vi "acqComponentsInit.vi"(1 "sCMOS init":cluster{"init":i16, "sCMOS handle":u32}, 2 "XY stage":T5, 3 "Z stage":T4, 4 "Filter wheel init":cluster{"FW Handle":u32, "init?":i16}, 6 "405 nm (aq)":bool=TRUE, 7 "405 nm filter":T3(ring), 8 "488 nm (aq)":bool=TRUE, 9 "488 nm filter":T3(ring)=enum."525/50 [FITC]", 10 "561 nm (aq)":bool=TRUE, 11 "561 nm filter":T3(ring)=enum."605/70 [Cy3]", 12 "642 nm (aq)":bool=TRUE, 13 "642 nm filter":T3(ring)=enum."665/LP [Cy5]") -> (15 "initializedLasers":T1(array[cluster]), 16 "Initialized filters":T2(array[ring])=[enum."460/36 [DAPI]", enum."525/50 [FITC]", enum."605/70 [Cy3]", enum."665/LP [Cy5]"], 17 "correctCompInit?":i32)   [LabVIEW 2015]
panel:
  in  "LSFM_3 lasers":T1(array[cluster])=[{"Component ID"="405nm", "COM Port"="COM14", "Type "=enum."omicronLuxX", "init"=1}, {"Component ID"="488nm", "COM Port"="COM4", "Type "=enum."omicronLuxX", "init"=1}, {"Component ID"="561nm", "COM Port"="COM27", "Type "=enum."coherentObis", "init"=1}, {"Component ID"="642nm", "COM Port"="COM12", "Type "=enum."omicronLuxX", "init"=1}]
  out "Correct lasers init?":i32=1
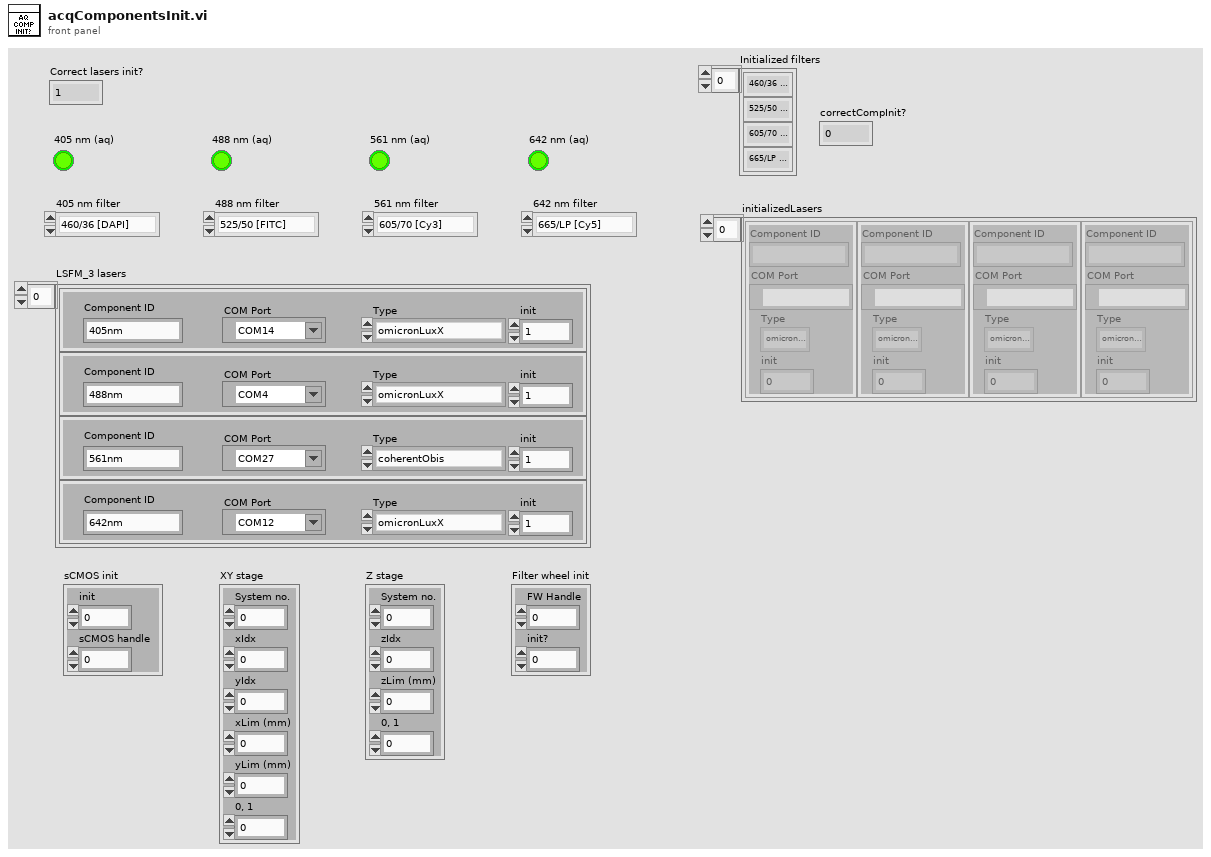
[diagram p1: front panel]
types:
  T1 = cluster{"Component ID":string, "COM Port":refnum<visa-resource-name>, "Type ":enum16{"omicronLuxX", "coherentObis"}, "init":i16}[]
  T2 = enum16{"460/36 [DAPI]", "525/50 [FITC]", "605/70 [Cy3]", "665/LP [Cy5]", "Empty-1", "Empty-2"}[]
  T3 = enum16{"460/36 [DAPI]", "525/50 [FITC]", "605/70 [Cy3]", "665/LP [Cy5]", "Empty-1", "Empty-2"}
  T4 = cluster{"System no.":i32, "zIdx":i32, "zLim (mm)":dbl, "0, 1":i16}
  T5 = cluster{"System no.":i32, "xIdx":i32, "yIdx":i32, "xLim (mm)":dbl, "yLim (mm)":dbl, "0, 1":i16}
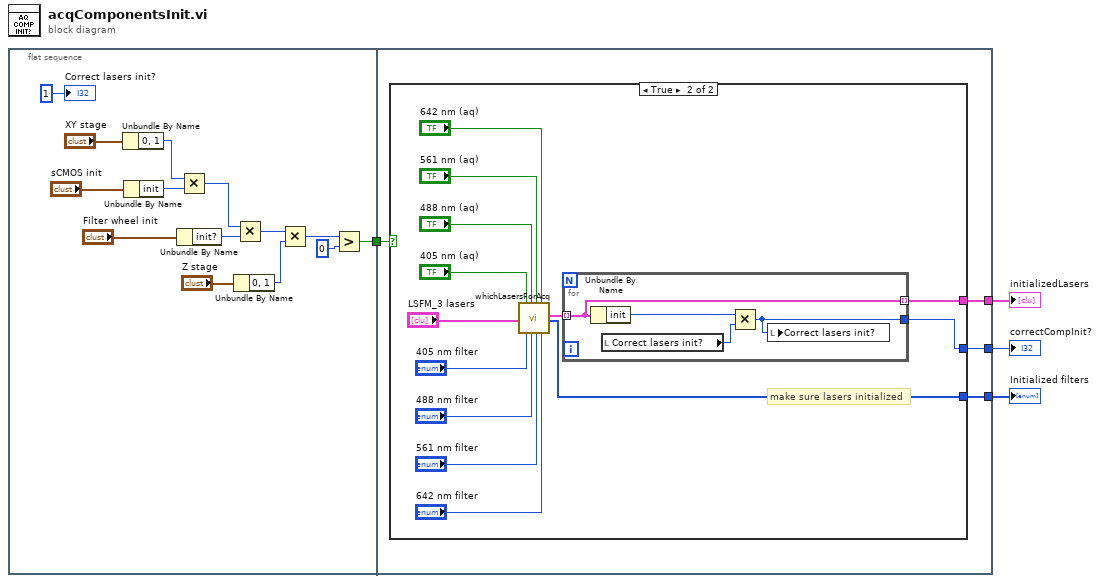
[diagram p0: block diagram]
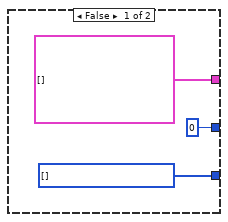
[diagram p2: hidden frame]
diagram:
  n1 = flat-sequence {
    tunnel: [w5] -> w1
    tunnel: [w22] -> w4
    tunnel: [w21] -> w3
    tunnel: [w20] -> w2
    tunnel: w1 -> [w19]
    frame #0 {
      n2 = Unbundle By Name("XY stage") -> ("0, 1"=w13:i16)
      n3 = Unbundle By Name("sCMOS init") -> ("init"=w12:i16)
      n4 = Unbundle By Name("Filter wheel init") -> ("init?"=w10:i16)
      n5 = Multiply(x=w13, y=w12) -> (x*y=w11:i16)
      n6 = Unbundle By Name("Z stage") -> ("0, 1"=w8:i16)
      n7 = Multiply(x=w11, y=w10) -> (x*y=w9:i16)
      n8 = Multiply(x=w9, y=w8) -> (x*y=w6:i16)
      n9 = Greater?(x=w6, y=0) -> (0:w5:bool)
      "Correct lasers init?" <- 1 ("Correct lasers init?")
    }
    frame #1 {
      n10 = case shown="True" w19 {
        tunnel: [0 w28] -> w22
        tunnel: [T1 [] w27] -> w21
        tunnel: [w23 w26] -> w20
        frame False {
          w23 = T2 [] items=["460/36 [DAPI]", "525/50 [FITC]", "605/70 [Cy3]", "665/LP [Cy5]", "Empty-1", "Empty-2"] ("Array 2")
        }
        frame True {
          # "make sure lasers initialized"
          n11 = call "whichLasersForAcq.vi"("LSFM_3 lasers"="LSFM_3 lasers", "405 nm (aq)"="405 nm (aq)", "405 nm filter"="405 nm filter", "488 nm (aq)"="488 nm (aq)", "488 nm filter"="488 nm filter", "561 nm (aq)"="561 nm (aq)", "561 nm filter"="561 nm filter", "642 nm (aq)"="642 nm (aq)", "642 nm filter"="642 nm filter") -> ("Initialized lasers"=w38:T1, "initializedFilters"=w26:T2)  [unwired: 9 in]
          n12 = for {
            tunnel: w38 -> [w39] mode=indexing
            tunnel: [w40] -> w28
            tunnel: [w39] -> w27 mode=indexing
            n13 = Unbundle By Name(w39) -> ("init"=w42:i16)
            n14 = local read "Correct lasers init?"() -> (w41:i32)
            n15 = Multiply(x=w42, y=w41) -> (x*y=w40:i32)
            n16 = local write "Correct lasers init?"(w40) -> ()
          }
        }
      }
    }
  }
  "correctCompInit?" <- w4
  "initializedLasers" <- w3
  "Initialized filters" <- w2
